vi "LJM read open config.vi"(0 "Working Directory":path, 5 "filename":string="ljlogm_open.cfg") -> (4 "DeviceType":string="LJM_dtANY", 6 "ConnectionType":string="LJM_ctANY", 8 "Identifier":string="LJM_idANY", 10 "Good Open Config":bool, 15 "error out":errorcluster)   [LabVIEW 2022 SP3]
uses:
  <vilib>/Utility/config.llb/Read Key (String).vi
  <vilib>/Utility/config.llb/NI_LVConfig.lvlib
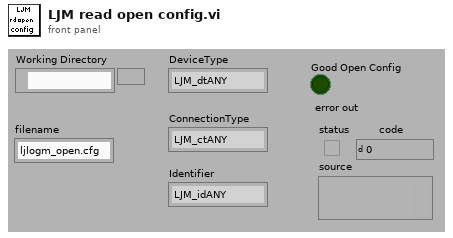
[diagram p1: front panel]
types:
  T1 = typedef "NI_LVConfig.lvlib/Config Data RefNum.ctl" = refnum<k1>
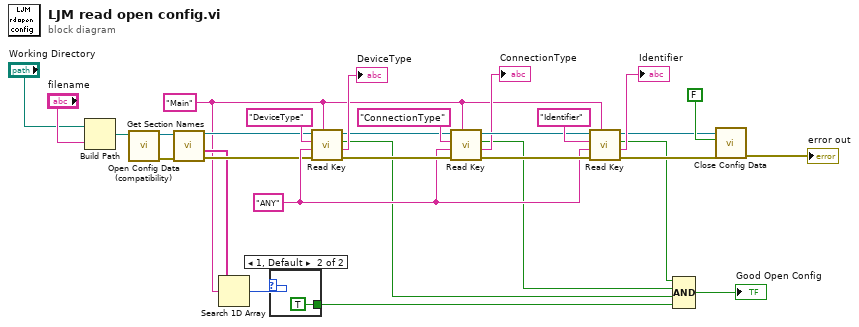
[diagram p0: block diagram]
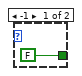
[diagram p2: hidden frame]
diagram:
  w14 = "ANY" ("Data File Prefix")
  w2 = "Main" ("section")
  n1 = Build Path(base path="Working Directory", name or relative path="filename") -> (appended path=w15:path)
  n2 = call <vilib>:"Open Config Data (compatibility).vi"("configuration file path"=w15) -> ("error out"=w7:errorcluster, "refnum"=w6:T1)  [unwired: 8 in, 1 out]
  n3 = call <vilib>:"Get Section Names.vi"("error in (no error)"=w7, "refnum"=w6) -> ("error out"=w4:errorcluster, "section names"=w3:string[], "refnum out"=w5:T1)  [unwired: 7 in]
  n4 = Search 1D Array(1D array=w3, element=w2) -> (index of element=w9:i32)  [unwired: 1 in]
  n5 = case shown="1, Default" w9 {
    tunnel: [FALSE TRUE] -> w8
    frame -1 {
    }
    frame 1, Default {
    }
  }
  n6 = call-poly <vilib>:"Read Key.vi"("section"=w2, "error in (no error)"=w4, "default value"=w14, "key"="DeviceType", "refnum"=w5) -> ("error out"=w23:errorcluster, "value"=→"DeviceType":string, "found?"=w12:bool, "refnum out"=w22:T1)  [unwired: 3 in]
  n7 = call-poly <vilib>:"Read Key.vi"("section"=w2, "error in (no error)"=w23, "default value"=w14, "key"="ConnectionType", "refnum"=w22) -> ("error out"=w21:errorcluster, "value"=→"ConnectionType":string, "found?"=w11:bool, "refnum out"=w20:T1)  [unwired: 3 in]
  n8 = call-poly <vilib>:"Read Key.vi"("section"=w2, "error in (no error)"=w21, "default value"=w14, "key"="Identifier", "refnum"=w20) -> ("error out"=w16:errorcluster, "value"=→"Identifier":string, "found?"=w10:bool, "refnum out"=w17:T1)  [unwired: 3 in]
  n9 = Compound Arithmetic op=AND(w10, w11, w12, w8) -> (→"Good Open Config":bool)
  n10 = call <vilib>:"Close Config Data.vi"("error in (no error)"=w16, "write file if changed (T)"=FALSE ("write configuration file? (F)"), "refnum"=w17) -> ("error out"=→"error out":errorcluster)  [unwired: 7 in, 1 out]
